vi "Right Cargo Bay 2.vi"   [LabVIEW 2018]
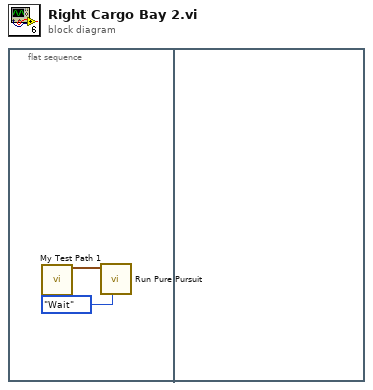
[diagram p0: block diagram]
diagram:
  n1 = flat-sequence {
    frame #0 {
      n2 = call "My Test Path 1.vi"() -> ("path"=w1:cluster{"X":dbl, "Y":dbl}[])  [unwired: 15 in]
      n3 = call "Run Pure Pursuit.vi"("Synchronication"=enum16{"Start", "Wait"}."Wait", "Path"=w1) -> ()  [unwired: 9 in, 1 out]
    }
    frame #1 {
    }
  }
